vi "Select_Elevator_From_Fleet.vi"(8 "error in (no error)":errorcluster, 10 "Elevator in":T2, 11 "Elevator Fleet in":T1) -> (0 "error out":errorcluster, 1 "ID":i32, 2 "Elevator out":T2, 3 "Elevator Fleet out":T1)   [LabVIEW 2026]
uses:
  Controls/Door_Status_Enum.ctl
  Controls/Occupy_Status.ctl
  Controls/Floor_Status.ctl
  Controls/Motion_Status_Enum.ctl
  Controls/Car_Calls_Status.ctl
  Controls/Hall_Calls_Status.ctl
  Controls/Elevator_Status.ctl
  Controls/Elevator_Fleet.ctl
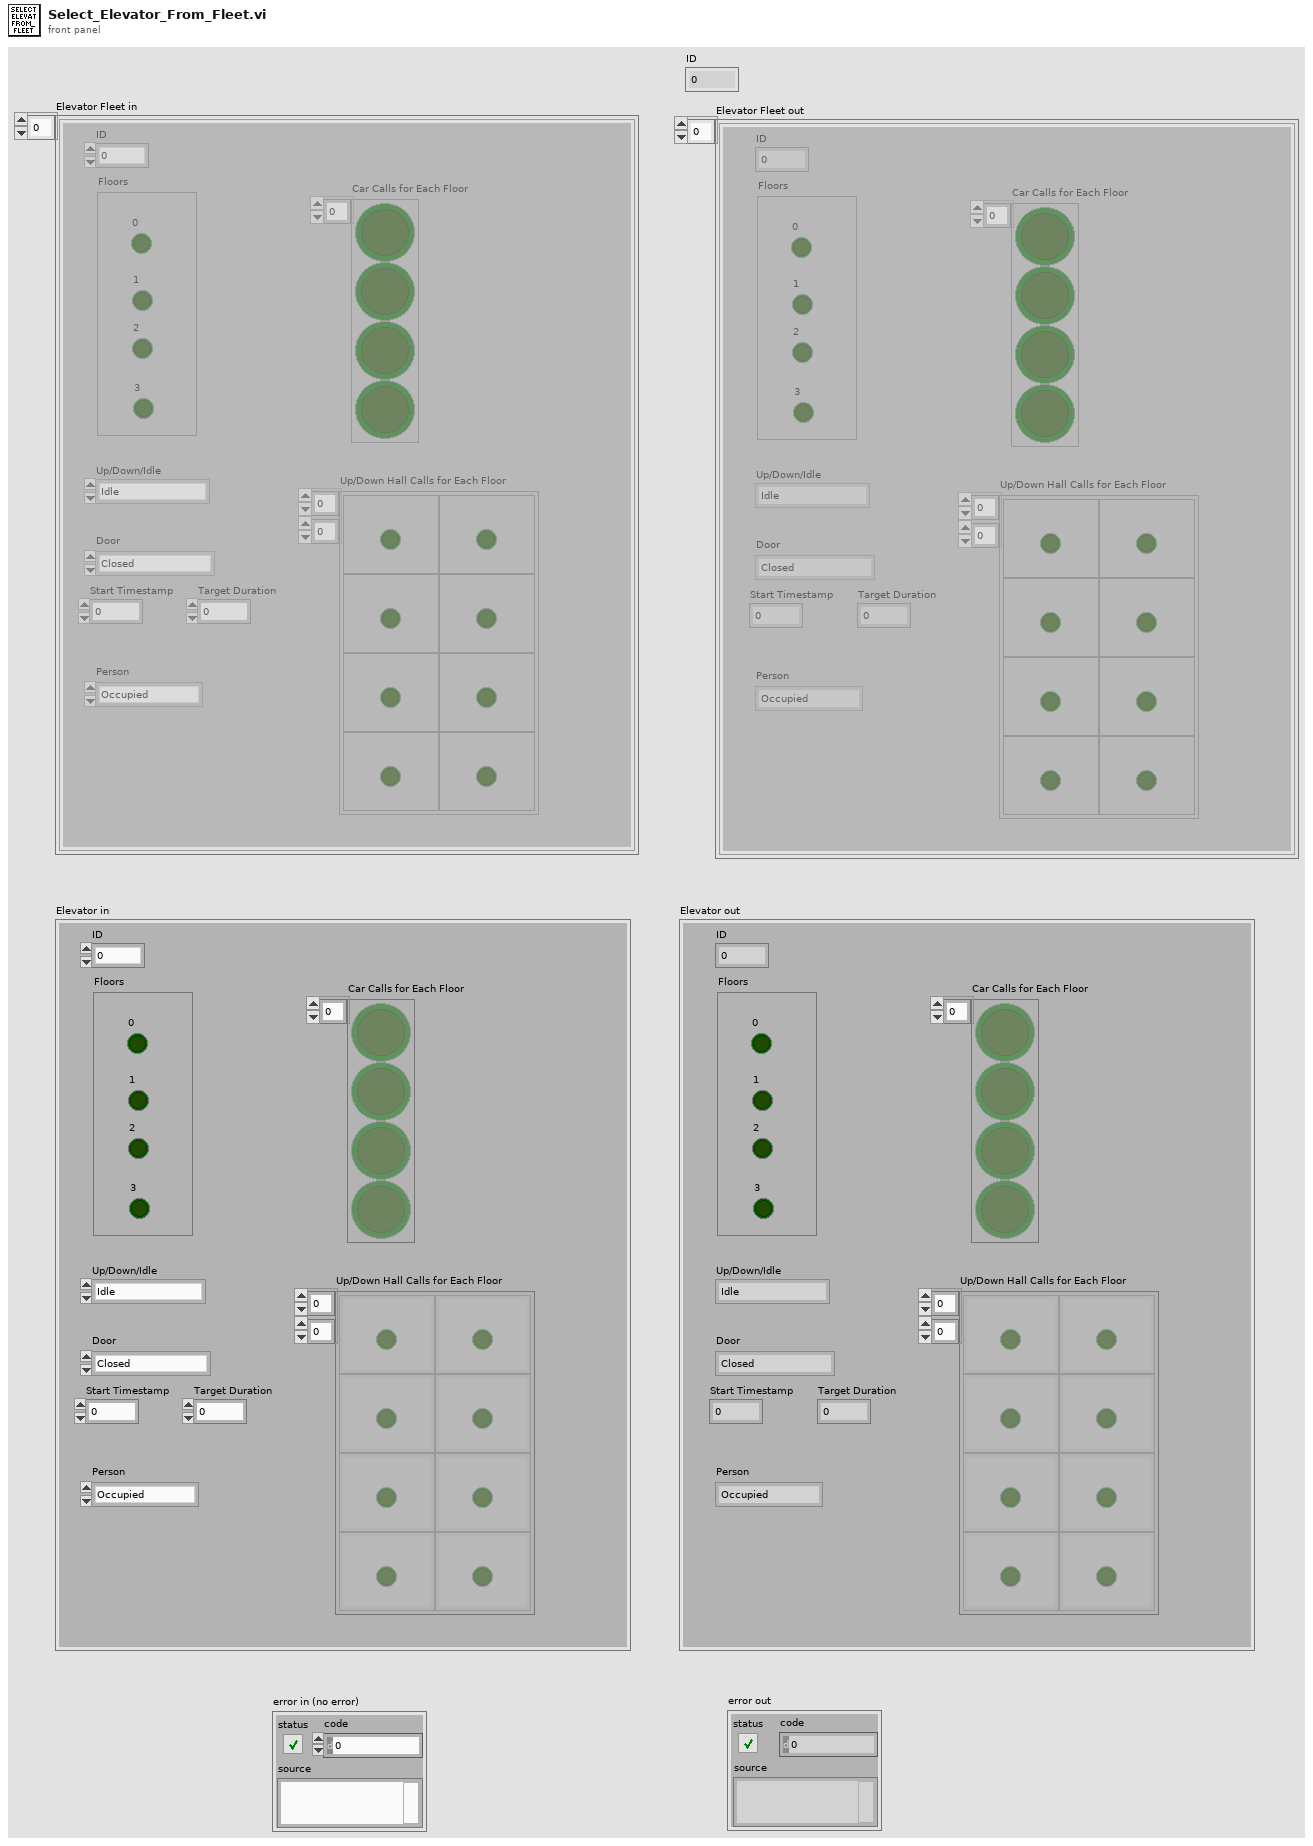
[diagram p1: front panel]
types:
  T1 = typedef "Elevator_Fleet.ctl" = T2[]
  T2 = typedef "Elevator_Status.ctl" = cluster{"Door":T3, "Person":T4, "Floors":T5, "Up/Down/Idle":T6, "Car Calls for Each Floor":T7, "Up/Down Hall Calls for Each Floor":T8, "ID":i32, "Start Timestamp":u32, "Target Duration":dbl}
  T3 = typedef "Door_Status_Enum.ctl" = enum16{"Closed", "Open", "Opening", "Closing"}
  T4 = typedef "Occupy_Status.ctl" = enum16{"Occupied", "Empty"}
  T5 = typedef "Floor_Status.ctl" = cluster{"0":bool, "1":bool, "2":bool, "3":bool}
  T6 = typedef "Motion_Status_Enum.ctl" = enum16{"Idle", "Up", "Down"}
  T7 = typedef "Car_Calls_Status.ctl" = bool[]
  T8 = typedef "Hall_Calls_Status.ctl" = cluster{bool}[][]
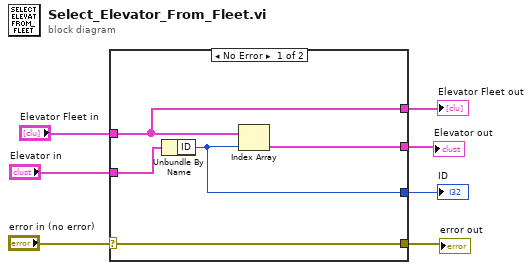
[diagram p0: block diagram]
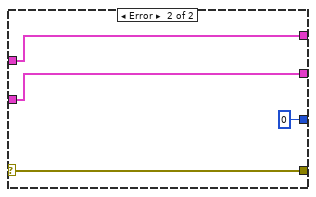
[diagram p2: hidden frame]
diagram:
  n1 = case shown="No Error" "error in (no error)" {
    selector: "error in (no error)" -> [w9 w16]
    tunnel: [w12 0 ("ID")] -> w7
    tunnel: "Elevator in" -> [w11 w15]
    tunnel: [w10 w15] -> w5
    tunnel: "Elevator Fleet in" -> [w8 w14]
    tunnel: [w9 w16] -> w2
    tunnel: [w8 w14] -> w1
    frame No Error {
      n2 = Unbundle By Name(w11) -> ("ID"=w12:i32)
      n3 = Index Array(array=w8, index=w12) -> (element=w10:T2)
    }
    frame Error {
    }
  }
  "ID" <- w7
  "Elevator out" <- w5
  "Elevator Fleet out" <- w1
  "error out" <- w2
